vi "set scans per acquisition.vi"(8 "error in (no error)":errorcluster, 11 "LineCCD in":refnum<class "LineCCD.lvclass">) -> (0 "error out":errorcluster, 3 "LineCCD out":refnum<class "LineCCD.lvclass">)   [LabVIEW 2012, in "LineCCD.lvclass"]
uses:
  LineCCD.lvclass
  <instrlib>/ALPHALAS CCD S Series/ALPHALAS CCD S Series.lvlib
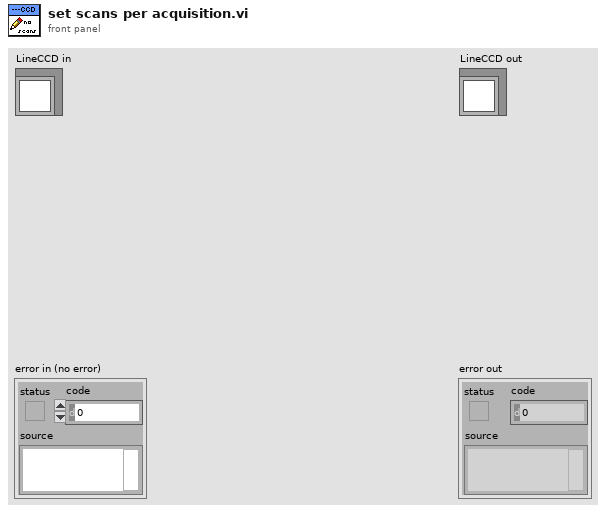
[diagram p1: front panel]
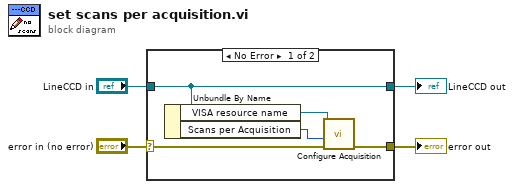
[diagram p0: block diagram]
diagram:
  n1 = case shown="No Error" "error in (no error)" {
    selector: "error in (no error)" -> [w8 w11]
    tunnel: [w7 w11] -> w3
    tunnel: [w6 w10] -> w1
    tunnel: "LineCCD in" -> [w6 w10]
    frame No Error {
      n2 = Unbundle By Name(w6) -> ("VISA resource name"=w9:refnum<visa-resource-name>, "Scans per Acquisition"=w5:u32)
      n3 = call <instrlib>:"Configure Acquisition.vi"("error in (no error)"=w8, "Scans per Acquisition (1)"=w5, "VISA resource name"=w9) -> ("error out"=w7:errorcluster)  [unwired: 7 in, 1 out]
    }
    frame Error {
    }
  }
  "error out" <- w3
  "LineCCD out" <- w1
